vi "Write Stderr.vi"(5 "Username":string, 6 "Password":string, 7 "Address":string, 8 "Error In":errorcluster) -> (0 "Error Out":errorcluster)   [LabVIEW 2018, in "Tests.lvlib" / "Channel.lvlib"]
uses:
  Channel.lvlib
  <vilib>/addons/_JKI Toolkits/Caraya/classes/Test/Test.lvclass
  <vilib>/addons/_JKI Toolkits/Caraya/classes/Assert/Assert.lvclass
  src/Toolkit/API/Channel/Channel.lvclass
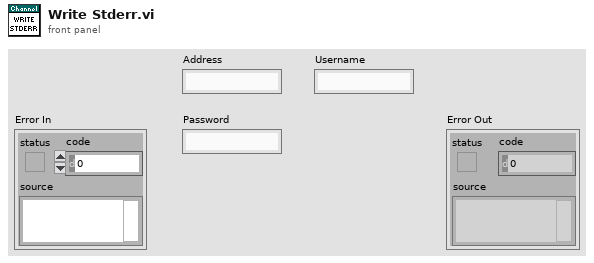
[diagram p1: front panel]
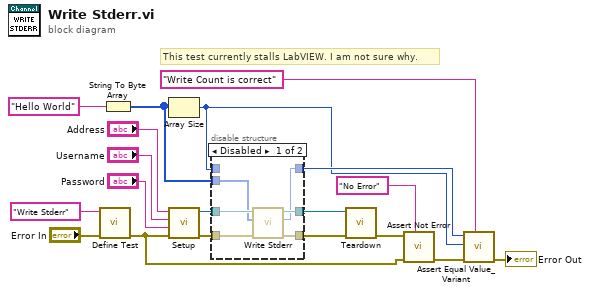
[diagram p0: block diagram]
diagram:
  # "This test currently stalls LabVIEW. I am not sure why."
  n1 = call <vilib>:"Define Test.vi"("error in (no error)"="Error In", "Label (VI Title)"="Write Stderr") -> ("error out"=w16:errorcluster)  [unwired: 9 in]
  n2 = String To Byte Array(string="Hello World") -> (unsigned byte array=w3:u8[])
  n3 = Array Size(array=w3) -> (size(s)=w1:i32)
  n4 = call "Setup.vi"("Error In"=w16, "Password"="Password", "Username"="Username", "Address"="Address") -> ("Error Out"=w11:errorcluster, "Channel"=w10:refnum<class "Channel.lvclass">)  [unwired: 6 in]
  n5 = disable-structure shown="Disabled" {
    disable-tunnel: w11 -> [w25 w27]
    disable-tunnel: w10 -> [w24 w28]
    disable-tunnel: [w23 w27] -> w8
    disable-tunnel: [w22 w28] -> w7
    disable-tunnel: [w21 w26] -> w4
    disable-tunnel: w3 -> [w20 _]
    disable-tunnel: w1 -> [_ w26]
    frame Disabled {
      n6 = call "Write Stderr.vi"("Error In"=w25, "Data"=w20, "Channel In"=w24) -> ("Error Out"=w23:errorcluster, "Write Count"=w21:u64, "Channel Out"=w22:refnum<class "Channel.lvclass">)  [unwired: 6 in]
    }
    frame Enabled {
    }
  }
  n7 = call "Teardown.vi"("Error In"=w8, "Channel"=w7) -> ("Error Out"=w12:errorcluster)  [unwired: 9 in]
  n8 = call <vilib>:"Assert Not Error.vi"("Label"="No Error", "error in (no error)"=w16, "Not Error?"=w12) -> ("error out"=w6:errorcluster)  [unwired: 8 in]
  n9 = call <vilib>:"Assert Equal Value_Variant.vi"("Label"="Write Count is correct", "error in (no error)"=w6, "Y"=w1, "X"=w4) -> ("error out"=→"Error Out":errorcluster)  [unwired: 7 in]
